vi "GeneratePhaseCUDAv3.vi"() -> ()   [LabVIEW 2019]
uses:
  <vilib>/imath/engines/lvmath2/RunTimeEngine/RangeToken/NIMS_Range.vi
  <instcachedir>/0/NIMS_Range_0856D726B6B24596B614846B21C682A9.lvgen/NIMS_Range_0856D726B6B24596B614846B21C682A9_001.vi
  <vilib>/imath/engines/lvmath2/RunTimeEngine/BuiltInFunctions/meshgrid2d/NIMS_meshgrid2d(V,V).vi
  <instcachedir>/0/NIMS_meshgrid2d(V,V)_3733343E1C554A708015CFB0432C6A59.lvgen/NIMS_meshgrid2d(V,V)_3733343E1C554A708015CFB0432C6A59_000.vi
  <vilib>/imath/engines/lvmath2/RunTimeEngine/ErrorHandling/NIMS_Create Error From Enums.vi
  <vilib>/imath/engines/lvmath2/RunTimeEngine/IndexRead/NIMS M($).vi
  <instcachedir>/0/NIMS M($)_82D1177398184AFB96A6AFB63C3C3F57.lvgen/NIMS M($)_82D1177398184AFB96A6AFB63C3C3F57_000.vi
  <vilib>/imathl/engines/lvmath/Functions/Error Handling/Create Error.vi
  <vilib>/imath/engines/lvmath2/RunTimeEngine/BuiltInFunctions/length/NIMS_length(GV).vi
  <instcachedir>/0/NIMS_length(GV)_08A3D13377FD4E4B96F5795FBF3698FA.lvgen/NIMS_length(GV)_08A3D13377FD4E4B96F5795FBF3698FA_000.vi
  <vilib>/imath/engines/lvmath2/RunTimeEngine/BuiltInFunctions/zeros/NIMS_V=zeros(I32,I32).vi
  <vilib>/imath/engines/lvmath2/RunTimeEngine/BuiltInFunctions/ones/NIMS_V=ones(I32,I32).vi
  <vilib>/imath/engines/lvmath2/RunTimeEngine/NodeEndStatement/NIMS_NodeEndStatement_Output.vi
  <instcachedir>/0/NIMS_NodeEndStatement_Output_53EC0D466D134D7ABD903AC30B43404B.lvgen/NIMS_NodeEndStatement_Output_53EC0D466D134D7ABD903AC30B43404B_005.vi
  <vilib>/imath/engines/lvmath2/RunTimeEngine/ErrorHandling/NIMS_Finalize Error.vi
  <instcachedir>/0/NIMS_NodeEndStatement_Output_53EC0D466D134D7ABD903AC30B43404B.lvgen/NIMS_NodeEndStatement_Output_53EC0D466D134D7ABD903AC30B43404B_011.vi
  <vilib>/imath/engines/lvmath2/RunTimeEngine/BuiltInFunctions/uint8/NIMS_uint8(real).vi
  <instcachedir>/0/NIMS_uint8(real)_CAA419FBB1354DA296C59E18C46DECF0.lvgen/NIMS_uint8(real)_CAA419FBB1354DA296C59E18C46DECF0_001.vi
  <vilib>/imath/engines/lvmath2/RunTimeEngine/BuiltInFunctions/mod/NIMS_mod_no_size_check.vi
  <instcachedir>/0/NIMS_mod_no_size_check_5393E3382FD241D281EEB71DA286C65B.lvgen/NIMS_mod_no_size_check_5393E3382FD241D281EEB71DA286C65B_004.vi
  <vilib>/imath/engines/lvmath2/RunTimeEngine/ArithmeticOperatorToken/NIMS_ArithmeticOperator_plus.vi
  <instcachedir>/0/NIMS_ArithmeticOperator_plus_A857F7369B7D4E138264023AAAB8243E.lvgen/NIMS_ArithmeticOperator_plus_A857F7369B7D4E138264023AAAB8243E_003.vi
  <instcachedir>/0/NIMS_meshgrid2d(V,V)_3733343E1C554A708015CFB0432C6A59.lvgen/NIMS_meshgrid2d(V,V)_3733343E1C554A708015CFB0432C6A59_005.vi
  PCIe16LabVIEWSDK/Interface.dll
  <vilib>/vision/NI_Vision_Development_Module.lvlib
panel:
  out "Total Phase":T1(plugin-control)
  in  "f [mm]":dbl=-300.0
  out "Fresnel Phase":T1(plugin-control)
  in  "Update SLM":bool
  out "Delay [ms] 2":dbl
  out "generatePhase Return 2":i32
  in  "I0":dbl=1.0
  in  "y0":i32
  in  "x0":i32
  in  "dy":i32=24
  in  "dx":i32=24
  in  "ny":i32=12
  in  "nx":i32=12
  in  "Generate":bool
  out "Y Array":sgl[](array[numeric])
  out "X Array":sgl[](array[numeric])
  out "board":i32
  in  "Start SLM":bool
  out "Board ID":i32
  out "# of Boards":i32
  in  "SLM":bool
  out "Delay [ms]":dbl
  out "startCuda Return":i32
  out "Init.":bool
  in  "N Iterations":i32=10
  out "N Pixels":i32
  out "SLM Size":i32
  in  "CUDA":bool
  out "stopCUDA Return":i32
  out "generatePhase Return":i32
  out "Path to CUDA DLL":path
  in  "Stop":bool
  out "CUDA Phase":T1(plugin-control)
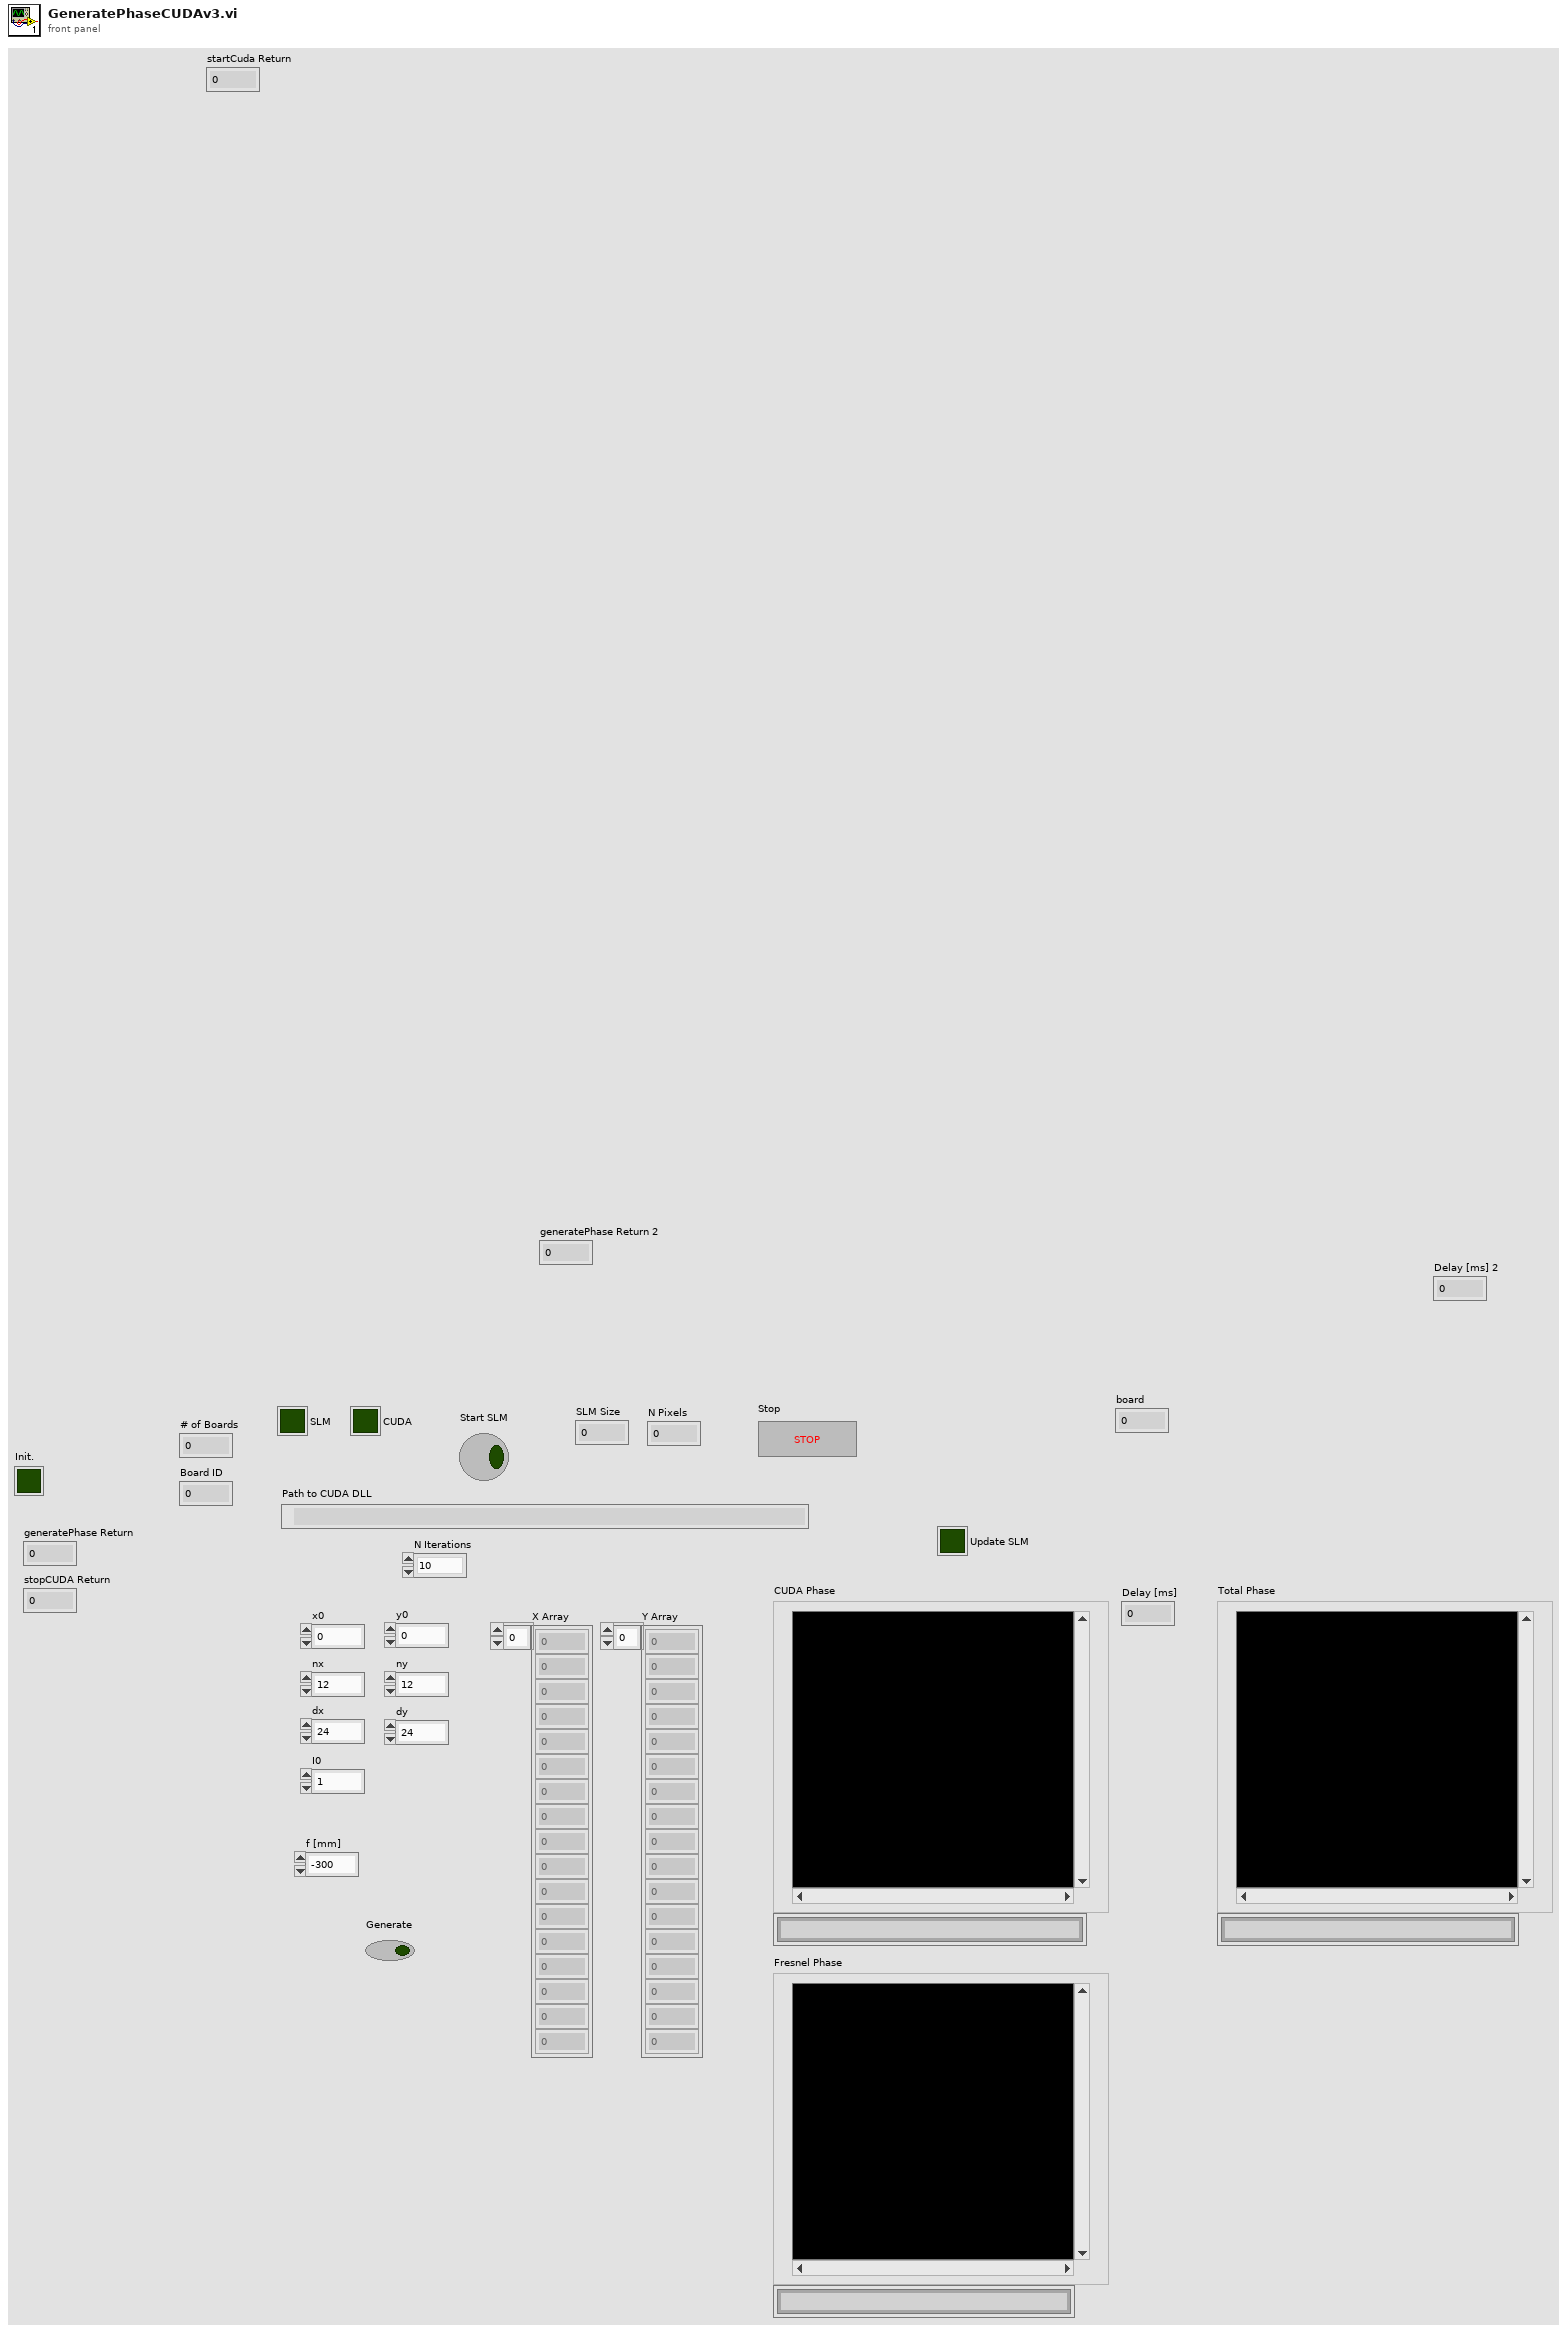
[diagram p1: front panel]
types:
  T1 = typedef "IMAQ Image.ctl" = refnum<image>
  T2 = typedef "Image Type" = u32
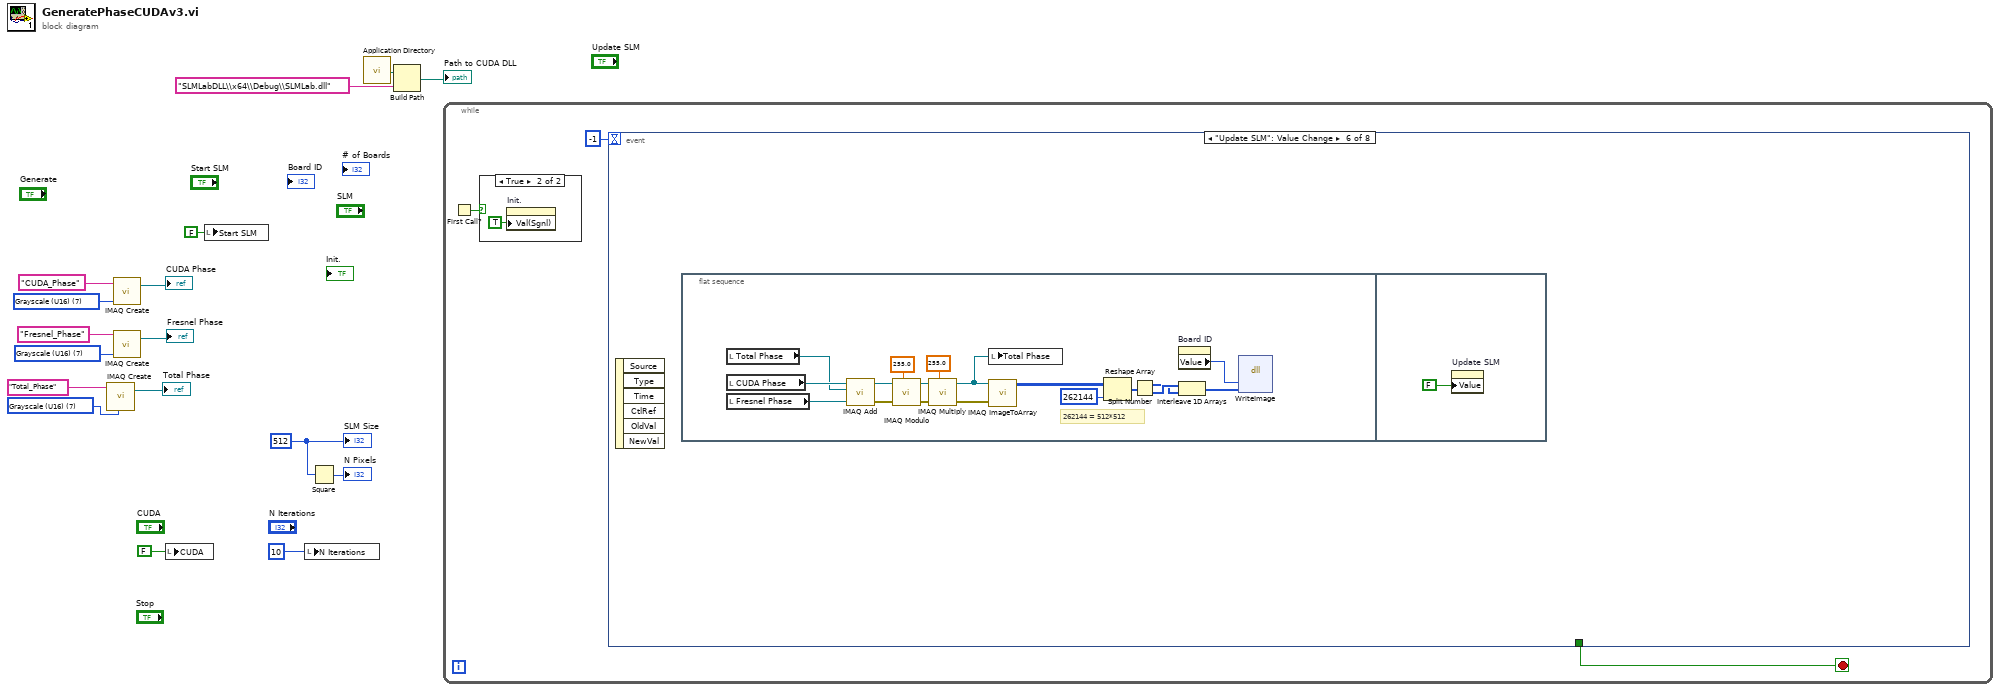
[diagram p0: block diagram]
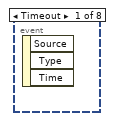
[diagram p3: hidden frame]
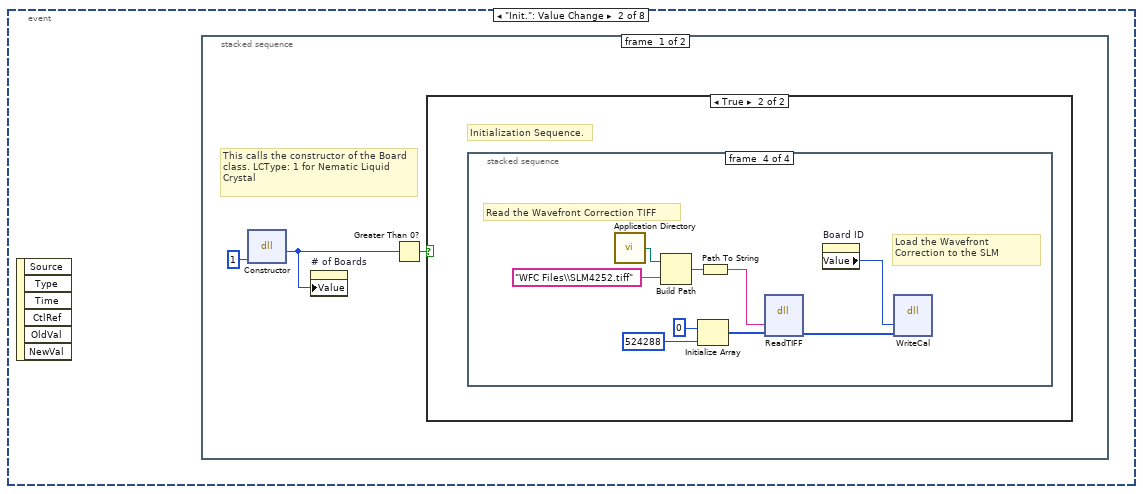
[diagram p4: hidden frame]
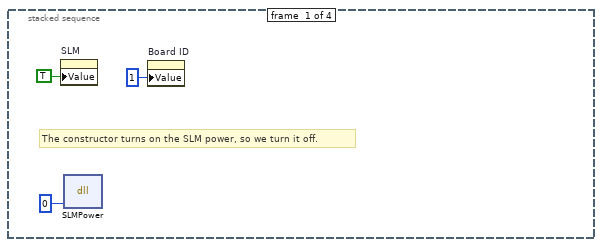
[diagram p6: hidden frame]
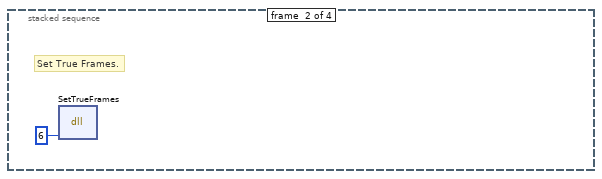
[diagram p7: hidden frame]
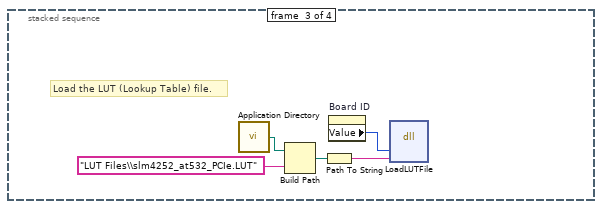
[diagram p8: hidden frame]
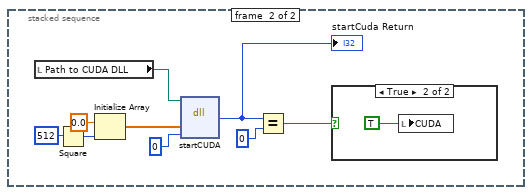
[diagram p9: hidden frame]
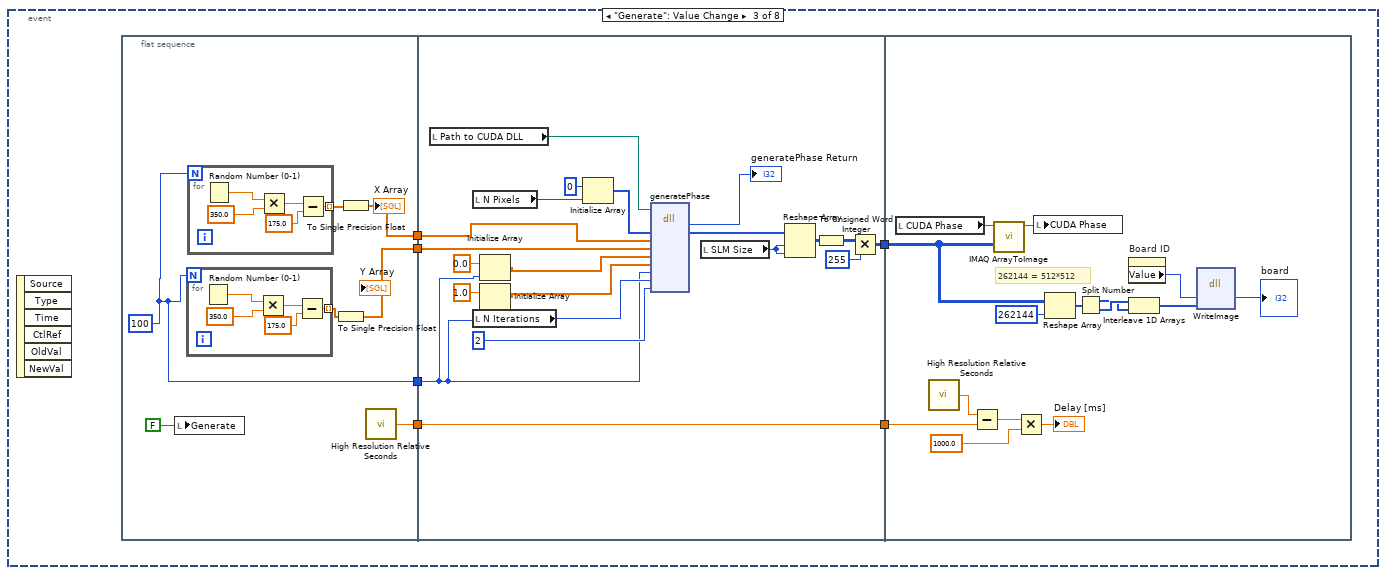
[diagram p11: hidden frame]
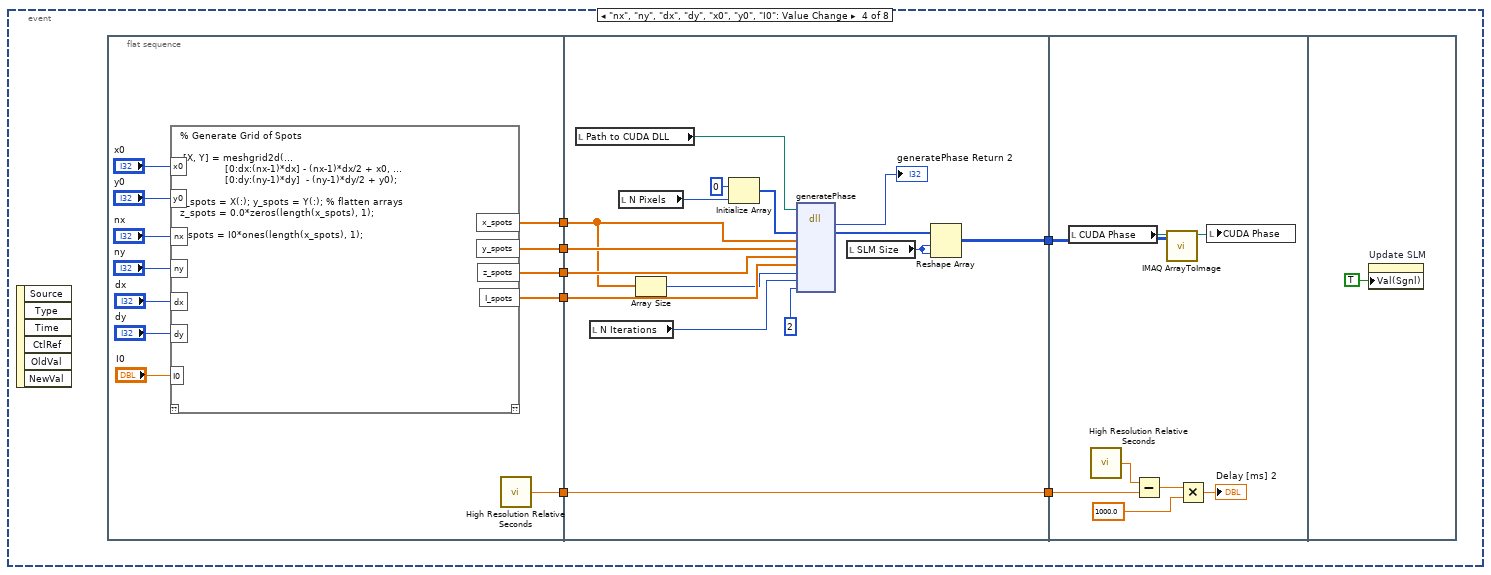
[diagram p12: hidden frame]
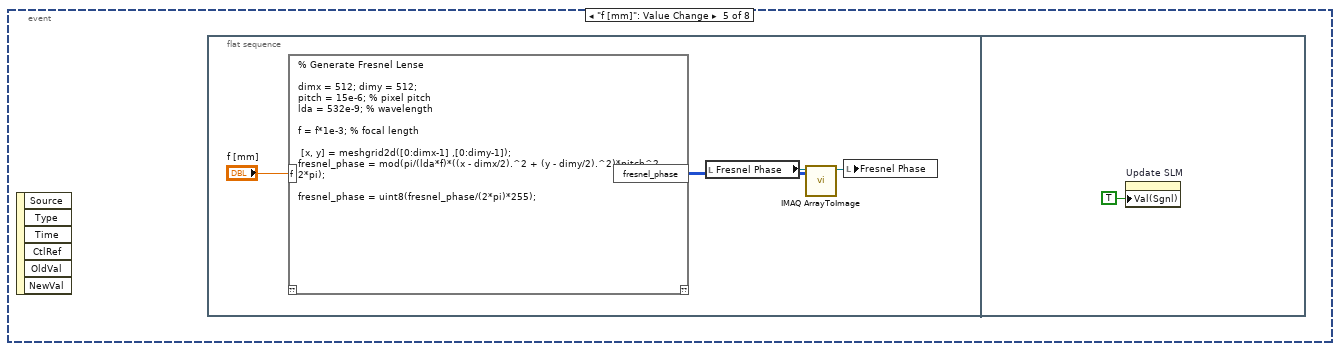
[diagram p13: hidden frame]
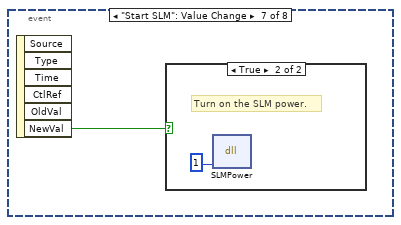
[diagram p14: hidden frame]
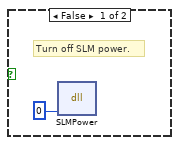
[diagram p15: hidden frame]
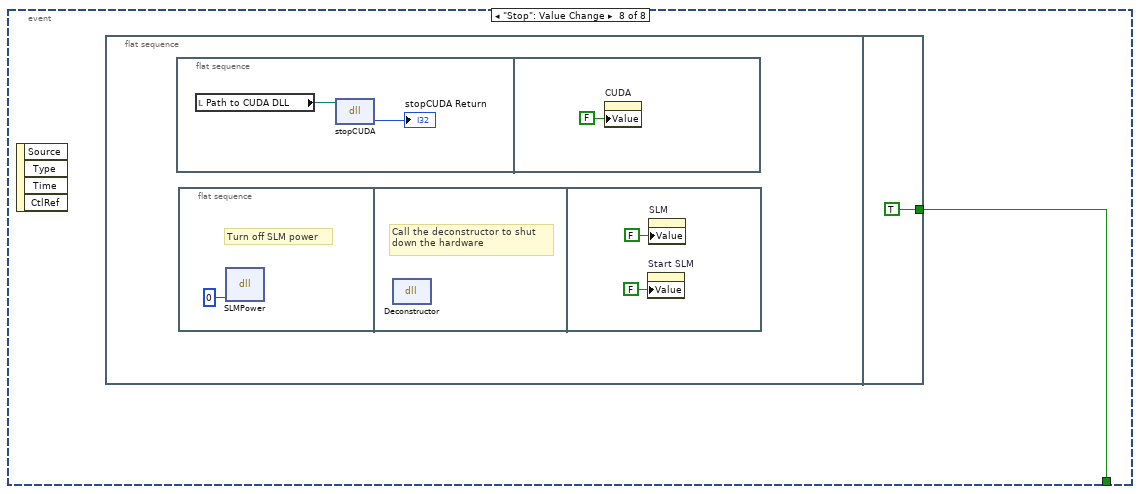
[diagram p16: hidden frame]
diagram:
  w1 = T2 7 items=["Grayscale (U8)", "Grayscale (I16)", "Grayscale (SGL)", "Complex (CSG)", "RGB (U32)", "HSL (U32)", "RGB (U64)", "Grayscale (U16)"] ("Image Type")
  w5 = T2 7 items=["Grayscale (U8)", "Grayscale (I16)", "Grayscale (SGL)", "Complex (CSG)", "RGB (U32)", "HSL (U32)", "RGB (U64)", "Grayscale (U16)"] ("Image Type")
  w9 = 512
  w16 = T2 7 items=["Grayscale (U8)", "Grayscale (I16)", "Grayscale (SGL)", "Complex (CSG)", "RGB (U32)", "HSL (U32)", "RGB (U64)", "Grayscale (U16)"] ("Image Type")
  n1 = call "IMAQ Create"("Image Name"="Total_Phase", "Image Type"=w1) -> ("New Image"=→"Total Phase":T1)  [unwired: 3 in, 1 out]
  n2 = call "IMAQ Create"("Image Name"="CUDA_Phase", "Image Type"=w16) -> ("New Image"=→"CUDA Phase":T1)  [unwired: 3 in, 1 out]
  n3 = call "IMAQ Create"("Image Name"="Fresnel_Phase", "Image Type"=w5) -> ("New Image"=→"Fresnel Phase":T1)  [unwired: 3 in, 1 out]
  n4 = local write "CUDA"(FALSE ("Update SLM")) -> ()
  n5 = local write "Start SLM"(FALSE ("Update SLM")) -> ()
  n6 = local write "N Iterations"(10) -> ()
  n7 = Square(x=w9) -> (x^2=→"N Pixels":i32)
  n8 = call <vilib>:"Application Directory.vi"() -> ("Application Directory"=w13:path)
  n9 = Build Path(base path=w13, name or relative path="SLMLabDLL\\x64\\Debug\\SLMLab.dll") -> (appended path=→"Path to CUDA DLL":path)
  n10 = while {
    stop <- w20 stop-if-true
    n11 = First Call?() -> (First Call?: T/F=w18:bool)
    n12 = case shown="True" w18 {
      frame False {
      }
      frame True {
        n13 = property on="Init." class="Bool (strict)"("Val(Sgnl)"=TRUE ("Value (Signaling)")) -> ()  [unwired: 2 in, 2 out]
      }
    }
    n14 = event shown="[5] \"Update SLM\": Value Change" {
      selector: _ -> [_ _ _ _ _ _ _ _]
      dyn-events: _ -> [_ _ _ _ _ _ _ _]
      timeout: -1 -> [_ _ _ _ _ _ _ _]
      tunnel: [_ _ _ _ _ _ _ w467] -> w20
      event Timeout {
        n15 = event-data() -> ()  [unwired: 1 in, 3 out]
      }
      event "Init.": Value Change {
        n16 = event-data() -> ()  [unwired: 1 in, 6 out]
        n17 = stacked-sequence {
          frame #0 {
            # "This calls the constructor of the Board class. LCType: 1 for Nematic Liquid Crystal"
            n18 = dll-call lib="C:/PCIe16LabVIEWSDK/Interface.dll" fn="Constructor"("LCType"=u8 1) -> ("return type"=w24:i32)  [unwired: 4 in, 2 out]
            n19 = property on="# of Boards" class="DigNum (strict)"("Value"=w24) -> ()  [unwired: 2 in, 2 out]
            n20 = Greater Than 0?(x=w24) -> (x > 0?=w23:bool)
            n21 = case shown="True" w23 {
              frame False {
              }
              frame True {
                # "Initialization Sequence."
                n22 = stacked-sequence {
                  frame #0 {
                    # "The constructor turns on the SLM power, so we turn it off."
                    n23 = property on="SLM" class="Bool (strict)"("Value"=TRUE ("SLM")) -> ()  [unwired: 2 in, 2 out]
                    n24 = dll-call lib="C:/PCIe16LabVIEWSDK/Interface.dll" fn="SLMPower"("PowerState"=0) -> ()  [unwired: 5 in, 2 out]
                    n25 = property on="Board ID" class="DigNum (strict)"("Value"=1 ("Board Number")) -> ()  [unwired: 2 in, 2 out]
                  }
                  frame #1 {
                    # "Set True Frames."
                    n26 = dll-call lib="C:/PCIe16LabVIEWSDK/Interface.dll" fn="SetTrueFrames"("TrueFrames"=6) -> ()  [unwired: 5 in, 2 out]
                  }
                  frame #2 {
                    # "Load the LUT (Lookup Table) file."
                    n27 = call <vilib>:"Application Directory.vi"() -> ("Application Directory"=w31:path)
                    n28 = Build Path(base path=w31, name or relative path="LUT Files\\slm4252_at532_PCIe.LUT") -> (appended path=w32:path)
                    n29 = Path To String(path=w32) -> (string=w29:string)
                    n30 = property on="Board ID" class="DigNum (strict)"() -> ("Value"=w33:i32)  [unwired: 2 in, 2 out]
                    n31 = dll-call lib="C:/PCIe16LabVIEWSDK/Interface.dll" fn="LoadLUTFile"("board"=w33, "LUTPath"=w29) -> ()  [unwired: 6 in, 2 out]
                  }
                  frame #3 {
                    # "Read the Wavefront Correction TIFF"
                    # "Load the Wavefront Correction to the SLM"
                    n32 = call <vilib>:"Application Directory.vi"() -> ("Application Directory"=w39:path)
                    n33 = Build Path(base path=w39, name or relative path="WFC Files\\SLM4252.tiff") -> (appended path=w40:path)
                    n34 = Initialize Array(u8 0, 524288) -> (w34:u8[])
                    n35 = Path To String(path=w40) -> (string=w37:string)
                    n36 = dll-call lib="C:/PCIe16LabVIEWSDK/Interface.dll" fn="ReadTIFF"("TiffPath"=w37, "Image"=w34) -> ("Image"=w42:u8[])  [unwired: 5 in, 2 out]
                    n37 = property on="Board ID" class="DigNum (strict)"() -> ("Value"=w41:i32)  [unwired: 2 in, 2 out]
                    n38 = dll-call lib="C:/PCIe16LabVIEWSDK/Interface.dll" fn="WriteCal"("board"=w41, "Image"=w42) -> ()  [unwired: 6 in, 2 out]
                  }
                }
              }
            }
          }
          frame #1 {
            n39 = local read "Path to CUDA DLL"() -> (w49:path)
            n40 = Square(x=512 ("dimension size")) -> (x^2=w51:i32)
            n41 = Initialize Array(sgl 0.0 ("element"), w51) -> (w50:sgl[])
            n42 = dll-call lib="?" fn="startCUDA"(path in=w49, "h_pSLMstart"=w50, "deviceID"=0) -> ("Rückgabetyp"=w48:i32)  [unwired: 4 in, 2 out]
            "startCuda Return" <- w48
            n43 = Equal?(x=w48, y=0) -> (x = y?=w47:bool)
            n44 = case shown="True" w47 {
              frame False {
              }
              frame True {
                n45 = local write "CUDA"(TRUE ("Update SLM")) -> ()
              }
            }
          }
        }
      }
      event "Generate": Value Change {
        n46 = event-data() -> ()  [unwired: 1 in, 6 out]
        n47 = flat-sequence {
          tunnel: [w65] -> w57
          tunnel: [w63] -> w55
          tunnel: [w61] -> w54
          tunnel: [w60] -> w53
          tunnel: [w88] -> w58
          tunnel: w57 -> [w88]
          tunnel: [w87] -> w56
          tunnel: w55 -> [w82]
          tunnel: w54 -> [w83]
          tunnel: w53 -> [w76]
          tunnel: w58 -> [w111]
          tunnel: w56 -> [w98]
          frame #0 {
            w60 = 100
            n48 = local write "Generate"(FALSE) -> ()
            n49 = for {
              N: w60 -> [_]
              tunnel: [w66] -> w62 mode=indexing
              n50 = Random Number (0-1)() -> (number: 0 to 1=w70:dbl)
              n51 = Multiply(x=w70, y=350.0) -> (x*y=w68:dbl)
              n52 = Subtract(x=w68, y=175.0) -> (x-y=w66:dbl)
            }
            n53 = for {
              N: w60 -> [_]
              tunnel: [w71] -> w64 mode=indexing
              n54 = Random Number (0-1)() -> (number: 0 to 1=w75:dbl)
              n55 = Multiply(x=w75, y=350.0) -> (x*y=w73:dbl)
              n56 = Subtract(x=w73, y=175.0) -> (x-y=w71:dbl)
            }
            n57 = To Single Precision Float(number=w62) -> (single precision float=w61:sgl[])
            "Y Array" <- w61
            n58 = To Single Precision Float(number=w64) -> (single precision float=w63:sgl[])
            "X Array" <- w63
            n59 = call <vilib>:"High Resolution Relative Seconds.vi"() -> ("relative seconds"=w65:dbl)
          }
          frame #1 {
            n60 = local read "Path to CUDA DLL"() -> (w93:path)
            n61 = local read "N Pixels"() -> (w94:i32)
            n62 = local read "N Iterations"() -> (w96:i32)
            n63 = Initialize Array(sgl 0.0 ("element"), w76) -> (w81:sgl[])
            n64 = Initialize Array(sgl 1.0 ("element"), w76) -> (w77:sgl[])
            n65 = Initialize Array(u8 0 ("element"), w94) -> (w92:u8[])
            n66 = dll-call lib="?" fn="generatePhase"(path in=w93, "h_pSLM_uint16"=w92, "x_spots"=w82, "y_spots"=w83, "z_spots"=w81, "I_spots"=w77, "N_spots"=w76, "N_interations"=w96, "method"=2) -> ("Return Value"=→"generatePhase Return":i32, "h_pSLM_uint16"=w91:u8[])  [unwired: 9 in, 2 out]
            n67 = local read "SLM Size"() -> (w95:i32)
            n68 = Reshape Array(w91, w95, w95) -> (w86:u8[][])
            n69 = To Unsigned Word Integer(number=w86) -> (unsigned 16bit integer=w85:u16[][])
            n70 = Multiply(x=w85, y=u16 255) -> (x*y=w87:u16[][])
          }
          frame #2 {
            # "262144 = 512*512"
            n71 = local read "CUDA Phase"() -> (w105:T1)
            n72 = call <vilib>:"High Resolution Relative Seconds.vi"() -> ("relative seconds"=w110:dbl)
            n73 = Subtract(x=w110, y=w111) -> (x-y=w109:dbl)
            n74 = call "IMAQ ArrayToImage"("Image Pixels (U16)"=w98, "Image"=w105) -> ("Image Out"=w106:T1)  [unwired: 8 in, 1 out]
            n75 = Multiply(x=w109, y=1000.0) -> (x*y=→"Delay [ms]":dbl)
            n76 = local write "CUDA Phase"(w106) -> ()
            n77 = Reshape Array(w98, 262144 ("dimension size")) -> (w103:u16[])
            n78 = Split Number(x=w103) -> (hi(x)=w100:u8[], lo(x)=w101:u8[])
            n79 = property on="Board ID" class="DigNum (strict)"() -> ("Value"=w104:i32)  [unwired: 2 in, 2 out]
            n80 = Interleave 1D Arrays(w101, w100) -> (w102:u8[])
            n81 = dll-call lib="C:/PCIe16LabVIEWSDK/Interface.dll" fn="WriteImage"("board"=w104, "Image"=w102) -> ("board"=→"board":i32)  [unwired: 5 in, 2 out]
          }
        }
      }
      event "nx", "ny", "dx", "dy", "x0", "y0", "I0": Value Change {
        n82 = event-data() -> ()  [unwired: 1 in, 6 out]
        n83 = flat-sequence {
          tunnel: [w130] -> w118
          tunnel: [w122] -> w117
          tunnel: [w121] -> w116
          tunnel: [w120] -> w115
          tunnel: [w119] -> w114
          tunnel: [w296] -> w113
          tunnel: w118 -> [w296]
          tunnel: w117 -> [w291]
          tunnel: w116 -> [w295]
          tunnel: w115 -> [w293]
          tunnel: w114 -> [w292]
          tunnel: [w289] -> w112
          tunnel: w113 -> [w312]
          tunnel: w112 -> [w305]
          frame #0 {
            n84 = mathscript code="% Generate Grid of Spots\n\n [X, Y] = meshgrid2d(...\n               [0:dx:(nx-1)*dx] - (nx-1)*dx/2 + x0, ...\n               [0:dy:(ny-1)*dy]  - (ny-1)*dy/2 + y0);\n\nx_spots = X(:); y_spots = Y(:); % flatten arrays\nz_spots = 0.0*zeros(length(x_spots), 1);\n\nI_spots = I0*ones(length(x_spots), 1);"("nx"="nx", "ny"="ny", "dx"="dx", "dy"="dy", "x0"="x0", "y0"="y0", "I0"="I0") -> ("x_spots"=w122:dbl[], "y_spots"=w121:dbl[], "I_spots"=w119:dbl[], "z_spots"=w120:dbl[])  [unwired: 1 in, 1 out]
            n85 = call <vilib>:"High Resolution Relative Seconds.vi"() -> ("relative seconds"=w130:dbl)
          }
          frame #1 {
            n86 = local read "Path to CUDA DLL"() -> (w301:path)
            n87 = local read "N Iterations"() -> (w304:i32)
            n88 = local read "N Pixels"() -> (w302:i32)
            n89 = Array Size(array=w291) -> (size(s)=w290:i32)
            n90 = Initialize Array(u8 0 ("element"), w302) -> (w300:u8[])
            n91 = dll-call lib="?" fn="generatePhase"(path in=w301, "h_pSLM_uint16"=w300, "x_spots"=w291, "y_spots"=w295, "z_spots"=w293, "I_spots"=w292, "N_spots"=w290, "N_interations"=w304, "method"=2) -> ("Return Value"=→"generatePhase Return 2":i32, "h_pSLM_uint16"=w299:u8[])  [unwired: 9 in, 2 out]
            n92 = local read "SLM Size"() -> (w303:i32)
            n93 = Reshape Array(w299, w303, w303) -> (w289:u8[][])
          }
          frame #2 {
            n94 = local read "CUDA Phase"() -> (w306:T1)
            n95 = call <vilib>:"High Resolution Relative Seconds.vi"() -> ("relative seconds"=w311:dbl)
            n96 = Subtract(x=w311, y=w312) -> (x-y=w310:dbl)
            n97 = call "IMAQ ArrayToImage"("Image Pixels (U16)"=w305, "Image"=w306) -> ("Image Out"=w307:T1)  [unwired: 8 in, 1 out]
            n98 = Multiply(x=w310, y=1000.0) -> (x*y=→"Delay [ms] 2":dbl)
            n99 = local write "CUDA Phase"(w307) -> ()
          }
          frame #3 {
            n100 = property on="Update SLM" class="Bool (strict)"("Val(Sgnl)"=TRUE ("Value (Signaling)")) -> ()  [unwired: 2 in, 2 out]
          }
        }
      }
      event "f [mm]": Value Change {
        n101 = event-data() -> ()  [unwired: 1 in, 6 out]
        n102 = flat-sequence {
          frame #0 {
            n103 = mathscript code="% Generate Fresnel Lense\n\ndimx = 512; dimy = 512;\npitch = 15e-6; % pixel pitch\nlda = 532e-9; % wavelength\n\nf = f*1e-3; % focal length\n\n [x, y] = meshgrid2d([0:dimx-1] ,[0:dimy-1]);\nfresnel_phase = mod(pi/(lda*f)*((x - dimx/2).^2 + (y - dimy/2).^2)*pitch^2 , 2*pi);\n\nfresnel_phase = uint8(fresnel_phase/(2*pi)*255);"("f"="f [mm]") -> ("fresnel_phase"=w314:u8[][])  [unwired: 1 in, 1 out]
            n104 = local read "Fresnel Phase"() -> (w315:T1)
            n105 = call "IMAQ ArrayToImage"("Image Pixels (U16)"=w314, "Image"=w315) -> ("Image Out"=w316:T1)  [unwired: 8 in, 1 out]
            n106 = local write "Fresnel Phase"(w316) -> ()
          }
          frame #1 {
            n107 = property on="Update SLM" class="Bool (strict)"("Val(Sgnl)"=TRUE ("Value (Signaling)")) -> ()  [unwired: 2 in, 2 out]
          }
        }
      }
      event "Update SLM": Value Change {
        n108 = event-data() -> ()  [unwired: 1 in, 6 out]
        n109 = flat-sequence {
          frame #0 {
            # "262144 = 512*512"
            n110 = local read "Total Phase"() -> (w447:T1)
            n111 = local read "CUDA Phase"() -> (w456:T1)
            n112 = local read "Fresnel Phase"() -> (w455:T1)
            n113 = call "IMAQ Add"("Image Src A"=w456, "Image Dst"=w447, "Image Src B"=w455) -> ("Image Dst Out"=w449:T1, "error out"=w453:errorcluster)  [unwired: 4 in]
            n114 = call "IMAQ Modulo"("Image Src A"=w449, "Constant"=255.0, "error in (no error)"=w453) -> ("Image Dst Out"=w448:T1, "error out"=w454:errorcluster)  [unwired: 4 in]
            n115 = call "IMAQ Multiply"("Image Src A"=w448, "Constant"=255.0) -> ("Image Dst Out"=w446:T1)  [unwired: 5 in, 1 out]
            n116 = local write "Total Phase"(w446) -> ()
            n117 = call "IMAQ ImageToArray"("error in (no error)"=w454, "Image"=w446) -> ("Image Pixels (U16)"=w452:u16[][])  [unwired: 2 in, 4 out]
            n118 = Reshape Array(w452, 262144 ("dimension size")) -> (w461:u16[])
            n119 = Split Number(x=w461) -> (hi(x)=w458:u8[], lo(x)=w459:u8[])
            n120 = property on="Board ID" class="DigNum (strict)"() -> ("Value"=w462:i32)  [unwired: 2 in, 2 out]
            n121 = Interleave 1D Arrays(w459, w458) -> (w460:u8[])
            n122 = dll-call lib="C:/PCIe16LabVIEWSDK/Interface.dll" fn="WriteImage"("board"=w462, "Image"=w460) -> ()  [unwired: 6 in, 2 out]
          }
          frame #1 {
            n123 = property on="Update SLM" class="Bool (strict)"("Value"=FALSE) -> ()  [unwired: 2 in, 2 out]
          }
        }
      }
      event "Start SLM": Value Change {
        n124 = event-data() -> ("NewVal"=w464:bool)  [unwired: 1 in, 5 out]
        n125 = case shown="True" w464 {
          frame False {
            # "Turn off SLM power."
            n126 = dll-call lib="C:/PCIe16LabVIEWSDK/Interface.dll" fn="SLMPower"("PowerState"=0) -> ()  [unwired: 5 in, 2 out]
          }
          frame True {
            # "Turn on the SLM power."
            n127 = dll-call lib="C:/PCIe16LabVIEWSDK/Interface.dll" fn="SLMPower"("PowerState"=1) -> ()  [unwired: 5 in, 2 out]
          }
        }
      }
      event "Stop": Value Change {
        n128 = event-data() -> ()  [unwired: 1 in, 4 out]
        n129 = flat-sequence {
          tunnel: [TRUE] -> w467
          frame #0 {
            n130 = flat-sequence {
              frame #0 {
                n131 = local read "Path to CUDA DLL"() -> (w468:path)
                n132 = dll-call lib="?" fn="stopCUDA"(path in=w468) -> ("Return Value"=→"stopCUDA Return":i32)  [unwired: 2 in, 2 out]
              }
              frame #1 {
                n133 = property on="CUDA" class="Bool (strict)"("Value"=FALSE ("SLM")) -> ()  [unwired: 2 in, 2 out]
              }
            }
            n134 = flat-sequence {
              frame #0 {
                # "Turn off SLM power"
                n135 = dll-call lib="C:/PCIe16LabVIEWSDK/Interface.dll" fn="SLMPower"("PowerState"=0) -> ()  [unwired: 5 in, 2 out]
              }
              frame #1 {
                # "Call the deconstructor to shut \ndown the hardware"
                n136 = dll-call lib="C:/PCIe16LabVIEWSDK/Interface.dll" fn="Deconstructor"() -> ()  [unwired: 4 in, 2 out]
              }
              frame #2 {
                n137 = property on="Start SLM" class="Bool (strict)"("Value"=FALSE ("SLM")) -> ()  [unwired: 2 in, 2 out]
                n138 = property on="SLM" class="Bool (strict)"("Value"=FALSE ("SLM")) -> ()  [unwired: 2 in, 2 out]
              }
            }
          }
          frame #1 {
          }
        }
      }
    }
  }
  "SLM Size" <- w9
